vi "Inficon 32 Bit Data.vi"(7 "Gas Type":enum16{"Natural Gas", "Propane Gas"}(ring), 8 "Error In":errorcluster, 10 "Inficon Data Input":T3={"Gross Heating Value, Vol (Real, Dry)"=65535.0, "Nitrogen Component Normalized Mole % (Dry)"=8.0, "Methane Component Normalized Mole % (Dry)"=69.0, "Carbon Dioxide Component Normalized Mole % (Dry)"=65535.0, "Ethane Component Normalized Mole % (Dry)"=65.0, "Propane Component Normalized Mole % (Dry)"=8.0, "i-Pentane Component Normalized Mole % (Dry)"=14.0, "i-Butane Component Normalized Mole % (Dry)"=66.0, "n-Butane Component Normalized Mole % (Dry)"=8.0, "n-Pentane Component Normalized Mole % (Dry)"=0.0, "Hexane Component Normalized Mole % (Dry)"=0.0, "Heptane Component Normalized Mole % (Dry)"=0.0, "Gross Wobbe Index, Real(Dry)"=0.0, "Relative Density, Real(Dry)"=40.0, "Propylene Component Normalized Mole % (Dry)"=0.0, "C4 Olefins Component Normalized Mole % (Dry)"=0.0, "Water Component Normalized Mole % (Dry)"=0.0}, 11 "Modbus master in":refnum<class "Modbus Master.lvclass">=refnum) -> (0 "Error Out":errorcluster, 2 "Inficon Data Output":T3, 3 "Modbus master out":refnum<class "Modbus Master.lvclass">, 5 "Text Array":string[][](array[string]))   [LabVIEW 2023]
uses:
  Type Definitions/Inficon Data.ctl
  <vilib>/NI/Modbus Library/API/Master/Modbus Master.lvclass
  <vilib>/NI/Modbus Library/Transmission Data Unit/IP/IP Data Unit.lvclass
  <vilib>/NI/Modbus Library/Master Function Definition/Master Function Definition.lvclass
  <vilib>/NI/Modbus Library/Network Protocol/Network Master/TCP/TCP Master.lvclass
  Type Definitions/Inficon Modbus Addresses.ctl
  Type Definitions/Inficon Modbus Addresses LP.ctl
panel:
  in  "Density LP":T1=126 items=["Gross Heating Value (Dry)"=100, "Ethane"=102, "Propane"=104, "Proplyene"=106, "i-Butane"=108, "n-butane"=110, "C4 Olefins"=112, "Water"=114, "Gross Wobbe Index (Dry)"=124, "Relative Density (Dry)"=126]
  in  "Wobbe LP":T1=124 items=["Gross Heating Value (Dry)"=100, "Ethane"=102, "Propane"=104, "Proplyene"=106, "i-Butane"=108, "n-butane"=110, "C4 Olefins"=112, "Water"=114, "Gross Wobbe Index (Dry)"=124, "Relative Density (Dry)"=126]
  in  "Water":T1=114 items=["Gross Heating Value (Dry)"=100, "Ethane"=102, "Propane"=104, "Proplyene"=106, "i-Butane"=108, "n-butane"=110, "C4 Olefins"=112, "Water"=114, "Gross Wobbe Index (Dry)"=124, "Relative Density (Dry)"=126]
  in  "C4":T1=112 items=["Gross Heating Value (Dry)"=100, "Ethane"=102, "Propane"=104, "Proplyene"=106, "i-Butane"=108, "n-butane"=110, "C4 Olefins"=112, "Water"=114, "Gross Wobbe Index (Dry)"=124, "Relative Density (Dry)"=126]
  in  "n-Butane LP":T1=110 items=["Gross Heating Value (Dry)"=100, "Ethane"=102, "Propane"=104, "Proplyene"=106, "i-Butane"=108, "n-butane"=110, "C4 Olefins"=112, "Water"=114, "Gross Wobbe Index (Dry)"=124, "Relative Density (Dry)"=126]
  in  "i-Butane LP":T1=108 items=["Gross Heating Value (Dry)"=100, "Ethane"=102, "Propane"=104, "Proplyene"=106, "i-Butane"=108, "n-butane"=110, "C4 Olefins"=112, "Water"=114, "Gross Wobbe Index (Dry)"=124, "Relative Density (Dry)"=126]
  in  "Proplyene":T1=106 items=["Gross Heating Value (Dry)"=100, "Ethane"=102, "Propane"=104, "Proplyene"=106, "i-Butane"=108, "n-butane"=110, "C4 Olefins"=112, "Water"=114, "Gross Wobbe Index (Dry)"=124, "Relative Density (Dry)"=126]
  in  "Propane":T1=104 items=["Gross Heating Value (Dry)"=100, "Ethane"=102, "Propane"=104, "Proplyene"=106, "i-Butane"=108, "n-butane"=110, "C4 Olefins"=112, "Water"=114, "Gross Wobbe Index (Dry)"=124, "Relative Density (Dry)"=126]
  in  "Ethane":T1=102 items=["Gross Heating Value (Dry)"=100, "Ethane"=102, "Propane"=104, "Proplyene"=106, "i-Butane"=108, "n-butane"=110, "C4 Olefins"=112, "Water"=114, "Gross Wobbe Index (Dry)"=124, "Relative Density (Dry)"=126]
  in  "HHV LP":T1=100 items=["Gross Heating Value (Dry)"=100, "Ethane"=102, "Propane"=104, "Proplyene"=106, "i-Butane"=108, "n-butane"=110, "C4 Olefins"=112, "Water"=114, "Gross Wobbe Index (Dry)"=124, "Relative Density (Dry)"=126]
  in  "Density NG":T2=126 items=["Gross Heating Value (Dry)"=100, "Nitrogen"=102, "Methane"=104, "CO2"=106, "Ethane"=108, "Propane"=110, "i-Butane"=112, "n-Butane"=114, "i-Pentane"=116, "n-Pentane"=118, "Hexane"=120, "Heptane"=122, "Gross Wobbe Index (Dry)"=124, "Relative Density (Dry)"=126]
  in  "Wobbe NG":T2=124 items=["Gross Heating Value (Dry)"=100, "Nitrogen"=102, "Methane"=104, "CO2"=106, "Ethane"=108, "Propane"=110, "i-Butane"=112, "n-Butane"=114, "i-Pentane"=116, "n-Pentane"=118, "Hexane"=120, "Heptane"=122, "Gross Wobbe Index (Dry)"=124, "Relative Density (Dry)"=126]
  in  "Heptane":T2=122 items=["Gross Heating Value (Dry)"=100, "Nitrogen"=102, "Methane"=104, "CO2"=106, "Ethane"=108, "Propane"=110, "i-Butane"=112, "n-Butane"=114, "i-Pentane"=116, "n-Pentane"=118, "Hexane"=120, "Heptane"=122, "Gross Wobbe Index (Dry)"=124, "Relative Density (Dry)"=126]
  in  "Hexane":T2=120 items=["Gross Heating Value (Dry)"=100, "Nitrogen"=102, "Methane"=104, "CO2"=106, "Ethane"=108, "Propane"=110, "i-Butane"=112, "n-Butane"=114, "i-Pentane"=116, "n-Pentane"=118, "Hexane"=120, "Heptane"=122, "Gross Wobbe Index (Dry)"=124, "Relative Density (Dry)"=126]
  in  "n-Pentane":T2=118 items=["Gross Heating Value (Dry)"=100, "Nitrogen"=102, "Methane"=104, "CO2"=106, "Ethane"=108, "Propane"=110, "i-Butane"=112, "n-Butane"=114, "i-Pentane"=116, "n-Pentane"=118, "Hexane"=120, "Heptane"=122, "Gross Wobbe Index (Dry)"=124, "Relative Density (Dry)"=126]
  in  "i-Pentane":T2=116 items=["Gross Heating Value (Dry)"=100, "Nitrogen"=102, "Methane"=104, "CO2"=106, "Ethane"=108, "Propane"=110, "i-Butane"=112, "n-Butane"=114, "i-Pentane"=116, "n-Pentane"=118, "Hexane"=120, "Heptane"=122, "Gross Wobbe Index (Dry)"=124, "Relative Density (Dry)"=126]
  in  "n-Butane":T2=114 items=["Gross Heating Value (Dry)"=100, "Nitrogen"=102, "Methane"=104, "CO2"=106, "Ethane"=108, "Propane"=110, "i-Butane"=112, "n-Butane"=114, "i-Pentane"=116, "n-Pentane"=118, "Hexane"=120, "Heptane"=122, "Gross Wobbe Index (Dry)"=124, "Relative Density (Dry)"=126]
  in  "i-Butane":T2=112 items=["Gross Heating Value (Dry)"=100, "Nitrogen"=102, "Methane"=104, "CO2"=106, "Ethane"=108, "Propane"=110, "i-Butane"=112, "n-Butane"=114, "i-Pentane"=116, "n-Pentane"=118, "Hexane"=120, "Heptane"=122, "Gross Wobbe Index (Dry)"=124, "Relative Density (Dry)"=126]
  in  "Propane":T2=110 items=["Gross Heating Value (Dry)"=100, "Nitrogen"=102, "Methane"=104, "CO2"=106, "Ethane"=108, "Propane"=110, "i-Butane"=112, "n-Butane"=114, "i-Pentane"=116, "n-Pentane"=118, "Hexane"=120, "Heptane"=122, "Gross Wobbe Index (Dry)"=124, "Relative Density (Dry)"=126]
  in  "Ethane":T2=108 items=["Gross Heating Value (Dry)"=100, "Nitrogen"=102, "Methane"=104, "CO2"=106, "Ethane"=108, "Propane"=110, "i-Butane"=112, "n-Butane"=114, "i-Pentane"=116, "n-Pentane"=118, "Hexane"=120, "Heptane"=122, "Gross Wobbe Index (Dry)"=124, "Relative Density (Dry)"=126]
  in  "CO2":T2=106 items=["Gross Heating Value (Dry)"=100, "Nitrogen"=102, "Methane"=104, "CO2"=106, "Ethane"=108, "Propane"=110, "i-Butane"=112, "n-Butane"=114, "i-Pentane"=116, "n-Pentane"=118, "Hexane"=120, "Heptane"=122, "Gross Wobbe Index (Dry)"=124, "Relative Density (Dry)"=126]
  in  "CH4":T2=104 items=["Gross Heating Value (Dry)"=100, "Nitrogen"=102, "Methane"=104, "CO2"=106, "Ethane"=108, "Propane"=110, "i-Butane"=112, "n-Butane"=114, "i-Pentane"=116, "n-Pentane"=118, "Hexane"=120, "Heptane"=122, "Gross Wobbe Index (Dry)"=124, "Relative Density (Dry)"=126]
  in  "N":T2=102 items=["Gross Heating Value (Dry)"=100, "Nitrogen"=102, "Methane"=104, "CO2"=106, "Ethane"=108, "Propane"=110, "i-Butane"=112, "n-Butane"=114, "i-Pentane"=116, "n-Pentane"=118, "Hexane"=120, "Heptane"=122, "Gross Wobbe Index (Dry)"=124, "Relative Density (Dry)"=126]
  in  "HHV NG":T2=100 items=["Gross Heating Value (Dry)"=100, "Nitrogen"=102, "Methane"=104, "CO2"=106, "Ethane"=108, "Propane"=110, "i-Butane"=112, "n-Butane"=114, "i-Pentane"=116, "n-Pentane"=118, "Hexane"=120, "Heptane"=122, "Gross Wobbe Index (Dry)"=124, "Relative Density (Dry)"=126]
  # "Propane Gas"
  # "Natural Gas"
  # "Natural Gas"
  # "Propane"
  # "Natural Gas"
  # "Propane"
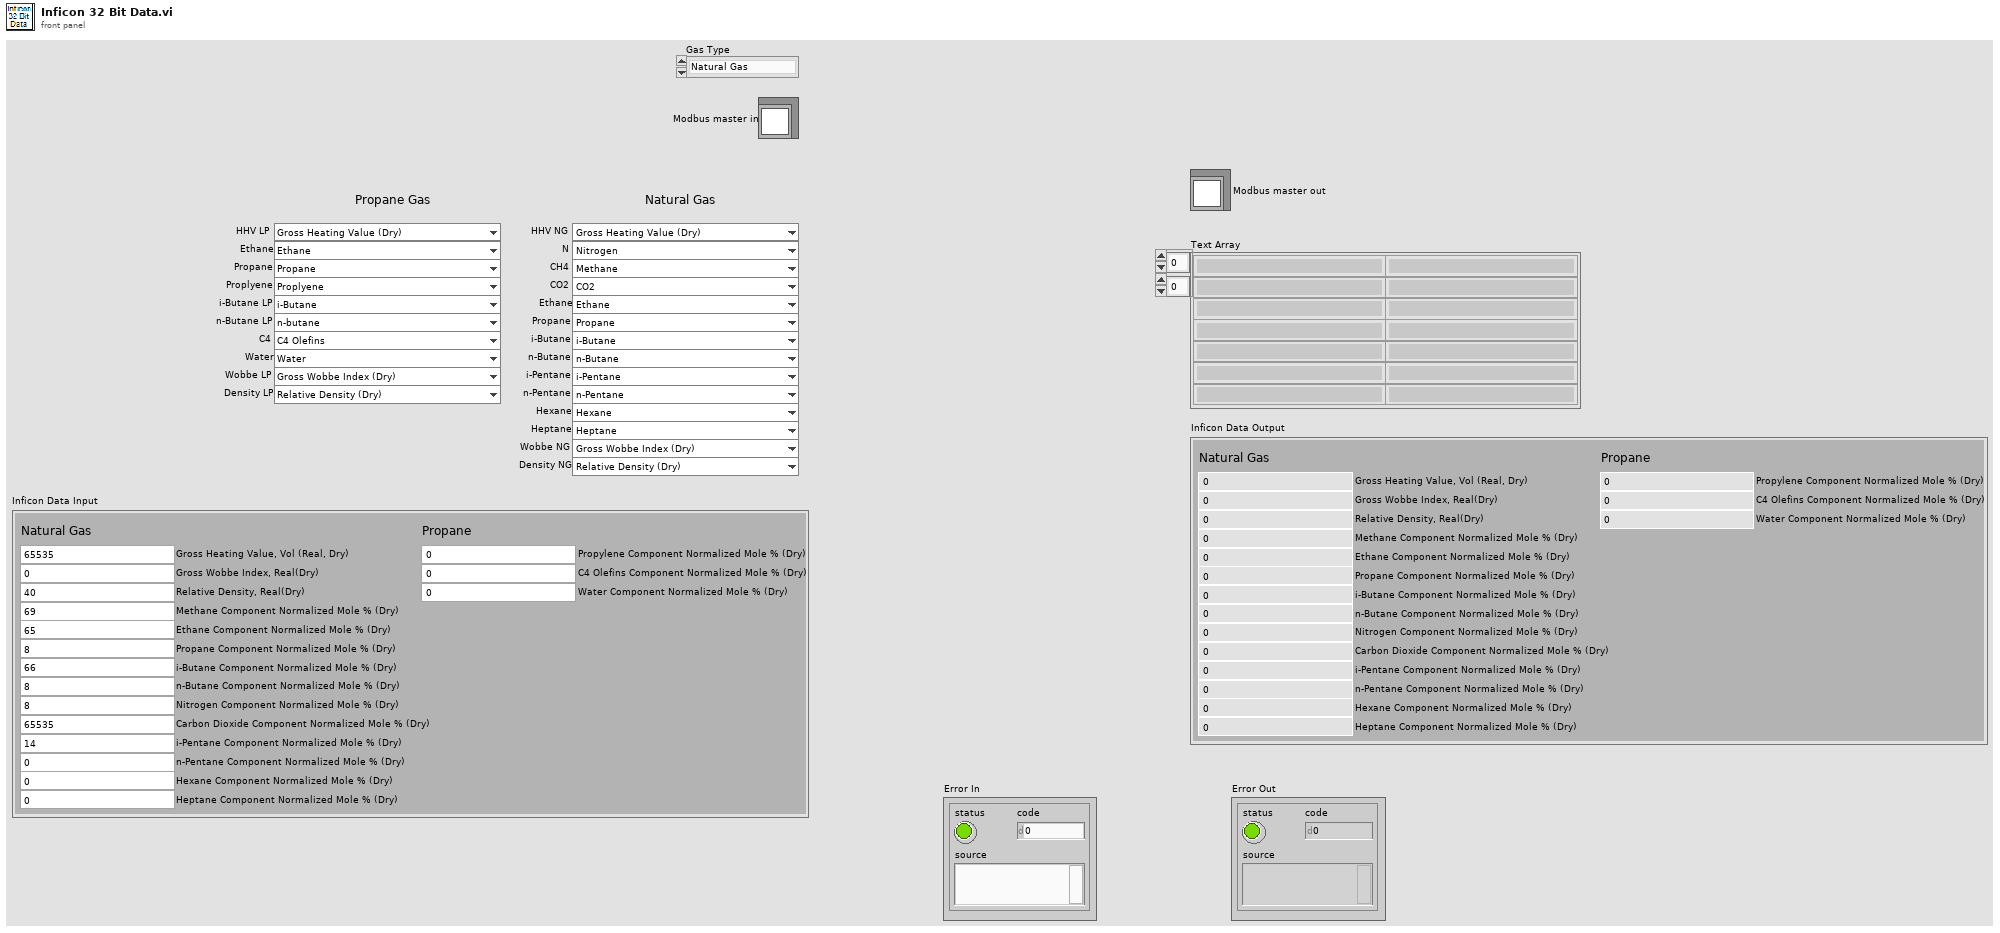
[diagram p1: front panel]
types:
  T1 = typedef "Inficon Modbus Addresses LP.ctl" = u16
  T2 = typedef "Inficon Modbus Addresses.ctl" = u16
  T3 = typedef "Inficon Data.ctl" = cluster{"Gross Heating Value, Vol (Real, Dry)":dbl, "Nitrogen Component Normalized Mole % (Dry)":dbl, "Methane Component Normalized Mole % (Dry)":dbl, "Carbon Dioxide Component Normalized Mole % (Dry)":dbl, "Ethane Component Normalized Mole % (Dry)":dbl, "Propane Component Normalized Mole % (Dry)":dbl, "i-Pentane Component Normalized Mole % (Dry)":dbl, "i-Butane Component Normalized Mole % (Dry)":dbl, "n-Butane Component Normalized Mole % (Dry)":dbl, "n-Pentane Component Normalized Mole % (Dry)":dbl, "Hexane Component Normalized Mole % (Dry)":dbl, "Heptane Component Normalized Mole % (Dry)":dbl, "Gross Wobbe Index, Real(Dry)":dbl, "Relative Density, Real(Dry)":dbl, "Propylene Component Normalized Mole % (Dry)":dbl, "C4 Olefins Component Normalized Mole % (Dry)":dbl, "Water Component Normalized Mole % (Dry)":dbl}
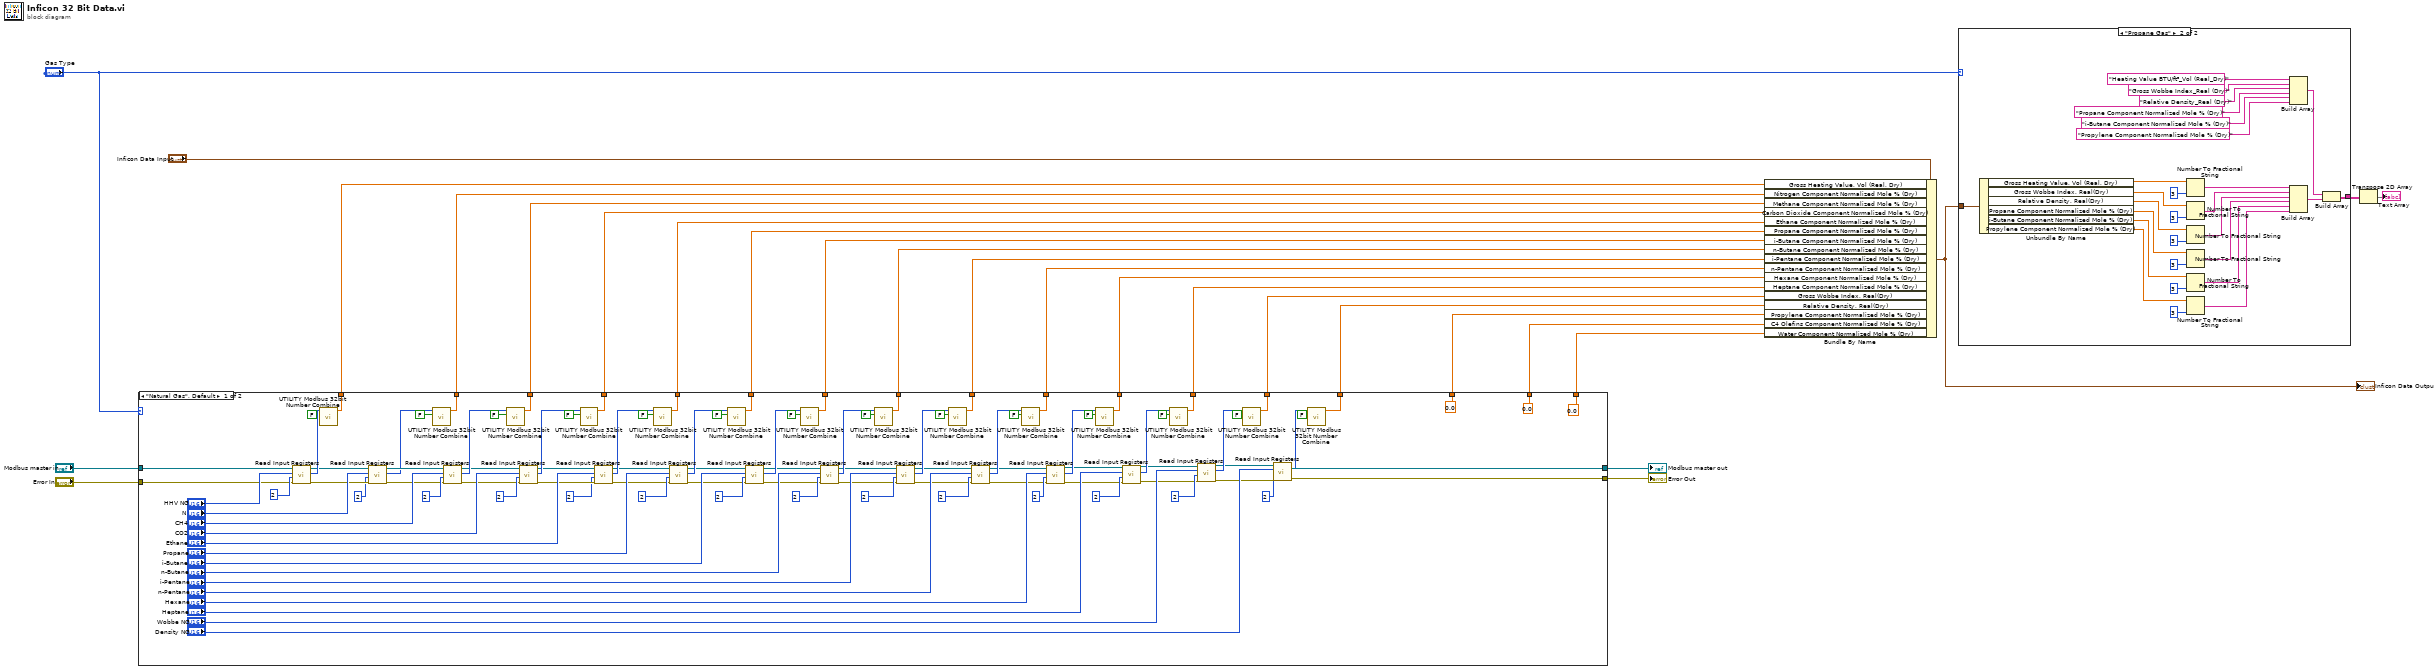
[diagram p0: block diagram]
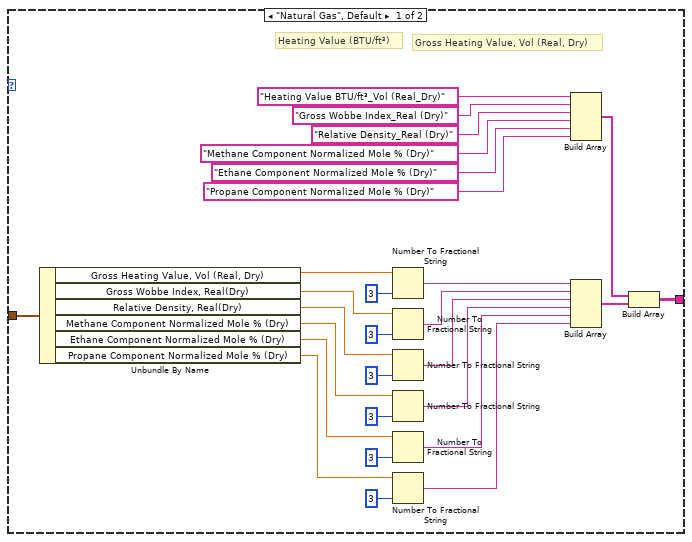
[diagram p2: hidden frame]
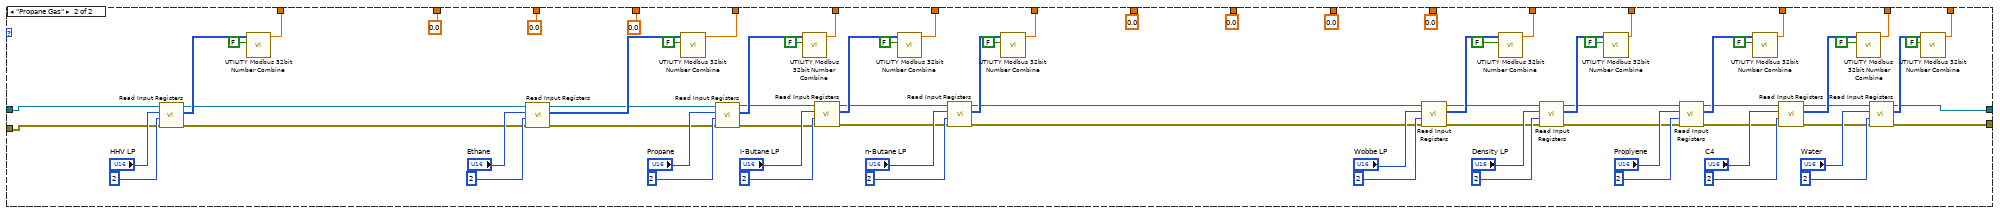
[diagram p3: hidden frame]
diagram:
  n1 = case shown="\"Natural Gas\", Default" "Gas Type" {
    tunnel: [w129 w202] -> w25
    tunnel: [w128 sgl 0.0 ("Data")] -> w24
    tunnel: [w127 sgl 0.0 ("Data")] -> w23
    tunnel: [w126 sgl 0.0 ("Data")] -> w22
    tunnel: [w125 w194] -> w21
    tunnel: [w124 sgl 0.0 ("Data")] -> w20
    tunnel: [w123 w190] -> w19
    tunnel: [w122 w184] -> w18
    tunnel: [w121 w179] -> w17
    tunnel: [w120 sgl 0.0 ("Data")] -> w16
    tunnel: "Modbus master in" -> [w111 w203]
    tunnel: "Error In" -> [w107 w204]
    tunnel: [w102 w130] -> w13
    tunnel: [w101 w131] -> w12
    tunnel: [w100 sgl 0.0 ("Data")] -> w11
    tunnel: [w99 sgl 0.0 ("Data")] -> w10
    tunnel: [w98 w171] -> w9
    tunnel: [w97 w165] -> w8
    tunnel: [0.0 ("Propylene Component Normalized Mole % (Dry)") w160] -> w4
    tunnel: [0.0 ("Propylene Component Normalized Mole % (Dry)") w151] -> w3
    tunnel: [0.0 ("Propylene Component Normalized Mole % (Dry)") w150] -> w2
    frame "Natural Gas", Default {
      n2 = call-dynamic "Read Input Registers.vi"("error in"=w107, "number of inputs"=u16 2 ("Quantity"), "starting address"="HHV NG", "Modbus master in"=w111) -> ("error out"=w103:errorcluster, "register values"=w108:u16[], "Modbus master out"=w105:refnum<class "Modbus Master.lvclass">)  [unwired: 5 in]
      n3 = call "UTILITY Modbus 32bit Number Combine.vi"("Swap Words"=FALSE, "Holding Registers"=w108) -> ("Data"=w129:sgl)  [unwired: 8 in, 1 out]
      n4 = call-dynamic "Read Input Registers.vi"("error in"=w103, "number of inputs"=u16 2 ("Quantity"), "starting address"="N", "Modbus master in"=w105) -> ("error out"=w58:errorcluster, "register values"=w59:u16[], "Modbus master out"=w60:refnum<class "Modbus Master.lvclass">)  [unwired: 5 in]
      n5 = call "UTILITY Modbus 32bit Number Combine.vi"("Swap Words"=FALSE, "Holding Registers"=w59) -> ("Data"=w128:sgl)  [unwired: 8 in, 1 out]
      n6 = call-dynamic "Read Input Registers.vi"("error in"=w58, "number of inputs"=u16 2 ("Quantity"), "starting address"="CH4", "Modbus master in"=w60) -> ("error out"=w85:errorcluster, "register values"=w91:u16[], "Modbus master out"=w87:refnum<class "Modbus Master.lvclass">)  [unwired: 5 in]
      n7 = call "UTILITY Modbus 32bit Number Combine.vi"("Swap Words"=FALSE, "Holding Registers"=w91) -> ("Data"=w127:sgl)  [unwired: 8 in, 1 out]
      n8 = call-dynamic "Read Input Registers.vi"("error in"=w85, "number of inputs"=u16 2 ("Quantity"), "starting address"="CO2", "Modbus master in"=w87) -> ("error out"=w84:errorcluster, "register values"=w90:u16[], "Modbus master out"=w86:refnum<class "Modbus Master.lvclass">)  [unwired: 5 in]
      n9 = call "UTILITY Modbus 32bit Number Combine.vi"("Swap Words"=FALSE, "Holding Registers"=w90) -> ("Data"=w126:sgl)  [unwired: 8 in, 1 out]
      n10 = call-dynamic "Read Input Registers.vi"("error in"=w84, "number of inputs"=u16 2 ("Quantity"), "starting address"="Ethane", "Modbus master in"=w86) -> ("error out"=w73:errorcluster, "register values"=w88:u16[], "Modbus master out"=w68:refnum<class "Modbus Master.lvclass">)  [unwired: 5 in]
      n11 = call "UTILITY Modbus 32bit Number Combine.vi"("Swap Words"=FALSE, "Holding Registers"=w88) -> ("Data"=w125:sgl)  [unwired: 8 in, 1 out]
      n12 = call-dynamic "Read Input Registers.vi"("error in"=w73, "number of inputs"=u16 2 ("Quantity"), "starting address"="Propane", "Modbus master in"=w68) -> ("error out"=w72:errorcluster, "register values"=w83:u16[], "Modbus master out"=w67:refnum<class "Modbus Master.lvclass">)  [unwired: 5 in]
      n13 = call "UTILITY Modbus 32bit Number Combine.vi"("Swap Words"=FALSE, "Holding Registers"=w83) -> ("Data"=w123:sgl)  [unwired: 8 in, 1 out]
      n14 = call-dynamic "Read Input Registers.vi"("error in"=w72, "number of inputs"=u16 2 ("Quantity"), "starting address"="i-Butane", "Modbus master in"=w67) -> ("error out"=w71:errorcluster, "register values"=w80:u16[], "Modbus master out"=w66:refnum<class "Modbus Master.lvclass">)  [unwired: 5 in]
      n15 = call "UTILITY Modbus 32bit Number Combine.vi"("Swap Words"=FALSE, "Holding Registers"=w80) -> ("Data"=w122:sgl)  [unwired: 8 in, 1 out]
      n16 = call-dynamic "Read Input Registers.vi"("error in"=w71, "number of inputs"=u16 2 ("Quantity"), "starting address"="n-Butane", "Modbus master in"=w66) -> ("error out"=w70:errorcluster, "register values"=w79:u16[], "Modbus master out"=w65:refnum<class "Modbus Master.lvclass">)  [unwired: 5 in]
      n17 = call "UTILITY Modbus 32bit Number Combine.vi"("Swap Words"=FALSE, "Holding Registers"=w79) -> ("Data"=w121:sgl)  [unwired: 8 in, 1 out]
      n18 = call-dynamic "Read Input Registers.vi"("error in"=w70, "number of inputs"=u16 2 ("Quantity"), "starting address"="i-Pentane", "Modbus master in"=w65) -> ("error out"=w69:errorcluster, "register values"=w76:u16[], "Modbus master out"=w64:refnum<class "Modbus Master.lvclass">)  [unwired: 5 in]
      n19 = call "UTILITY Modbus 32bit Number Combine.vi"("Swap Words"=FALSE, "Holding Registers"=w76) -> ("Data"=w120:sgl)  [unwired: 8 in, 1 out]
      n20 = call-dynamic "Read Input Registers.vi"("error in"=w69, "number of inputs"=u16 2 ("Quantity"), "starting address"="n-Pentane", "Modbus master in"=w64) -> ("error out"=w38:errorcluster, "register values"=w75:u16[], "Modbus master out"=w31:refnum<class "Modbus Master.lvclass">)  [unwired: 5 in]
      n21 = call "UTILITY Modbus 32bit Number Combine.vi"("Swap Words"=FALSE, "Holding Registers"=w75) -> ("Data"=w124:sgl)  [unwired: 8 in, 1 out]
      n22 = call-dynamic "Read Input Registers.vi"("error in"=w38, "number of inputs"=u16 2 ("Quantity"), "starting address"="Hexane", "Modbus master in"=w31) -> ("error out"=w37:errorcluster, "register values"=w47:u16[], "Modbus master out"=w32:refnum<class "Modbus Master.lvclass">)  [unwired: 5 in]
      n23 = call "UTILITY Modbus 32bit Number Combine.vi"("Swap Words"=FALSE, "Holding Registers"=w47) -> ("Data"=w100:sgl)  [unwired: 8 in, 1 out]
      n24 = call-dynamic "Read Input Registers.vi"("error in"=w37, "number of inputs"=u16 2 ("Quantity"), "starting address"="Heptane", "Modbus master in"=w32) -> ("error out"=w36:errorcluster, "register values"=w46:u16[], "Modbus master out"=w33:refnum<class "Modbus Master.lvclass">)  [unwired: 5 in]
      n25 = call "UTILITY Modbus 32bit Number Combine.vi"("Swap Words"=FALSE, "Holding Registers"=w46) -> ("Data"=w99:sgl)  [unwired: 8 in, 1 out]
      n26 = call-dynamic "Read Input Registers.vi"("error in"=w36, "number of inputs"=u16 2 ("Quantity"), "starting address"="Wobbe NG", "Modbus master in"=w33) -> ("error out"=w35:errorcluster, "register values"=w41:u16[], "Modbus master out"=w34:refnum<class "Modbus Master.lvclass">)  [unwired: 5 in]
      n27 = call "UTILITY Modbus 32bit Number Combine.vi"("Swap Words"=FALSE, "Holding Registers"=w41) -> ("Data"=w98:sgl)  [unwired: 8 in, 1 out]
      n28 = call-dynamic "Read Input Registers.vi"("error in"=w35, "number of inputs"=u16 2 ("Quantity"), "starting address"="Density NG", "Modbus master in"=w34) -> ("error out"=w102:errorcluster, "register values"=w30:u16[], "Modbus master out"=w101:refnum<class "Modbus Master.lvclass">)  [unwired: 5 in]
      n29 = call "UTILITY Modbus 32bit Number Combine.vi"("Swap Words"=FALSE, "Holding Registers"=w30) -> ("Data"=w97:sgl)  [unwired: 8 in, 1 out]
    }
    frame "Propane Gas" {
      n30 = call-dynamic "Read Input Registers.vi"("error in"=w204, "number of inputs"=u16 2 ("Quantity"), "starting address"="HHV LP", "Modbus master in"=w203) -> ("error out"=w149:errorcluster, "register values"=w207:u16[], "Modbus master out"=w148:refnum<class "Modbus Master.lvclass">)  [unwired: 5 in]
      n31 = call "UTILITY Modbus 32bit Number Combine.vi"("Swap Words"=FALSE, "Holding Registers"=w207) -> ("Data"=w202:sgl)  [unwired: 8 in, 1 out]
      n32 = call-dynamic "Read Input Registers.vi"("error in"=w149, "number of inputs"=u16 2 ("Quantity"), "starting address"="Ethane", "Modbus master in"=w148) -> ("error out"=w147:errorcluster, "register values"=w196:u16[], "Modbus master out"=w144:refnum<class "Modbus Master.lvclass">)  [unwired: 5 in]
      n33 = call "UTILITY Modbus 32bit Number Combine.vi"("Swap Words"=FALSE, "Holding Registers"=w196) -> ("Data"=w194:sgl)  [unwired: 8 in, 1 out]
      n34 = call-dynamic "Read Input Registers.vi"("error in"=w147, "number of inputs"=u16 2 ("Quantity"), "starting address"="Propane", "Modbus master in"=w144) -> ("error out"=w146:errorcluster, "register values"=w193:u16[], "Modbus master out"=w145:refnum<class "Modbus Master.lvclass">)  [unwired: 5 in]
      n35 = call "UTILITY Modbus 32bit Number Combine.vi"("Swap Words"=FALSE, "Holding Registers"=w193) -> ("Data"=w190:sgl)  [unwired: 8 in, 1 out]
      n36 = call-dynamic "Read Input Registers.vi"("error in"=w146, "number of inputs"=u16 2 ("Quantity"), "starting address"="i-Butane LP", "Modbus master in"=w145) -> ("error out"=w143:errorcluster, "register values"=w188:u16[], "Modbus master out"=w142:refnum<class "Modbus Master.lvclass">)  [unwired: 5 in]
      n37 = call "UTILITY Modbus 32bit Number Combine.vi"("Swap Words"=FALSE, "Holding Registers"=w188) -> ("Data"=w184:sgl)  [unwired: 8 in, 1 out]
      n38 = call-dynamic "Read Input Registers.vi"("error in"=w143, "number of inputs"=u16 2 ("Quantity"), "starting address"="n-Butane LP", "Modbus master in"=w142) -> ("error out"=w141:errorcluster, "register values"=w181:u16[], "Modbus master out"=w140:refnum<class "Modbus Master.lvclass">)  [unwired: 5 in]
      n39 = call "UTILITY Modbus 32bit Number Combine.vi"("Swap Words"=FALSE, "Holding Registers"=w181) -> ("Data"=w179:sgl)  [unwired: 8 in, 1 out]
      n40 = call-dynamic "Read Input Registers.vi"("error in"=w141, "number of inputs"=u16 2 ("Quantity"), "starting address"="Wobbe LP", "Modbus master in"=w140) -> ("error out"=w139:errorcluster, "register values"=w172:u16[], "Modbus master out"=w138:refnum<class "Modbus Master.lvclass">)  [unwired: 5 in]
      n41 = call "UTILITY Modbus 32bit Number Combine.vi"("Swap Words"=FALSE, "Holding Registers"=w172) -> ("Data"=w171:sgl)  [unwired: 8 in, 1 out]
      n42 = call-dynamic "Read Input Registers.vi"("error in"=w139, "number of inputs"=u16 2 ("Quantity"), "starting address"="Density LP", "Modbus master in"=w138) -> ("error out"=w137:errorcluster, "register values"=w169:u16[], "Modbus master out"=w136:refnum<class "Modbus Master.lvclass">)  [unwired: 5 in]
      n43 = call "UTILITY Modbus 32bit Number Combine.vi"("Swap Words"=FALSE, "Holding Registers"=w169) -> ("Data"=w165:sgl)  [unwired: 8 in, 1 out]
      n44 = call-dynamic "Read Input Registers.vi"("error in"=w137, "number of inputs"=u16 2 ("Quantity"), "starting address"="Proplyene", "Modbus master in"=w136) -> ("error out"=w134:errorcluster, "register values"=w162:u16[], "Modbus master out"=w135:refnum<class "Modbus Master.lvclass">)  [unwired: 5 in]
      n45 = call "UTILITY Modbus 32bit Number Combine.vi"("Swap Words"=FALSE, "Holding Registers"=w162) -> ("Data"=w160:sgl)  [unwired: 8 in, 1 out]
      n46 = call-dynamic "Read Input Registers.vi"("error in"=w134, "number of inputs"=u16 2 ("Quantity"), "starting address"="C4", "Modbus master in"=w135) -> ("error out"=w133:errorcluster, "register values"=w159:u16[], "Modbus master out"=w132:refnum<class "Modbus Master.lvclass">)  [unwired: 5 in]
      n47 = call "UTILITY Modbus 32bit Number Combine.vi"("Swap Words"=FALSE, "Holding Registers"=w159) -> ("Data"=w151:sgl)  [unwired: 8 in, 1 out]
      n48 = call-dynamic "Read Input Registers.vi"("error in"=w133, "number of inputs"=u16 2 ("Quantity"), "starting address"="Water", "Modbus master in"=w132) -> ("error out"=w130:errorcluster, "register values"=w153:u16[], "Modbus master out"=w131:refnum<class "Modbus Master.lvclass">)  [unwired: 5 in]
      n49 = call "UTILITY Modbus 32bit Number Combine.vi"("Swap Words"=FALSE, "Holding Registers"=w153) -> ("Data"=w150:sgl)  [unwired: 8 in, 1 out]
    }
  }
  "Error Out" <- w13
  "Modbus master out" <- w12
  n50 = Bundle By Name(cluster="Inficon Data Input", "Gross Heating Value, Vol (Real, Dry)"=w25, "Nitrogen Component Normalized Mole % (Dry)"=w24, "Methane Component Normalized Mole % (Dry)"=w23, "Carbon Dioxide Component Normalized Mole % (Dry)"=w22, "Ethane Component Normalized Mole % (Dry)"=w21, "Propane Component Normalized Mole % (Dry)"=w19, "i-Butane Component Normalized Mole % (Dry)"=w18, "n-Butane Component Normalized Mole % (Dry)"=w17, "i-Pentane Component Normalized Mole % (Dry)"=w16, "n-Pentane Component Normalized Mole % (Dry)"=w20, "Hexane Component Normalized Mole % (Dry)"=w11, "Heptane Component Normalized Mole % (Dry)"=w10, "Gross Wobbe Index, Real(Dry)"=w9, "Relative Density, Real(Dry)"=w8, "Propylene Component Normalized Mole % (Dry)"=w4, "C4 Olefins Component Normalized Mole % (Dry)"=w3, "Water Component Normalized Mole % (Dry)"=w2) -> (w7:T3)
  "Inficon Data Output" <- w7
  n51 = case shown="\"Propane Gas\"" "Gas Type" {
    tunnel: w7 -> [w236 w237]
    tunnel: [w229 w238] -> w6
    frame "Natural Gas", Default {
      # "Gross Heating Value, Vol (Real, Dry)"
      # "Heating Value (BTU/ft³)"
      n52 = Unbundle By Name(w236) -> ("Gross Heating Value, Vol (Real, Dry)"=w235:dbl, "Gross Wobbe Index, Real(Dry)"=w223:dbl, "Relative Density, Real(Dry)"=w222:dbl, "Methane Component Normalized Mole % (Dry)"=w221:dbl, "Ethane Component Normalized Mole % (Dry)"=w220:dbl, "Propane Component Normalized Mole % (Dry)"=w219:dbl)
      n53 = Number To Fractional String(number=w235, precision (6)=i16 3) -> (F-format string=w232:string)  [unwired: 2 in]
      n54 = Number To Fractional String(number=w223, precision (6)=i16 3) -> (F-format string=w218:string)  [unwired: 2 in]
      n55 = Number To Fractional String(number=w222, precision (6)=i16 3) -> (F-format string=w217:string)  [unwired: 2 in]
      n56 = Number To Fractional String(number=w221, precision (6)=i16 3) -> (F-format string=w216:string)  [unwired: 2 in]
      n57 = Number To Fractional String(number=w220, precision (6)=i16 3) -> (F-format string=w215:string)  [unwired: 2 in]
      n58 = Number To Fractional String(number=w219, precision (6)=i16 3) -> (F-format string=w214:string)  [unwired: 2 in]
      n59 = Build Array("Heating Value BTU/ft³_Vol (Real_Dry)", "Gross Wobbe Index_Real (Dry)", "Relative Density_Real (Dry)", "Methane Component Normalized Mole % (Dry)", "Ethane Component Normalized Mole % (Dry)", "Propane Component Normalized Mole % (Dry)") -> (w231:string[])
      n60 = Build Array(w232, w218, w217, w216, w215, w214) -> (w230:string[])
      n61 = Build Array(w231, w230) -> (w229:string[][])
    }
    frame "Propane Gas" {
      n62 = Unbundle By Name(w237) -> ("Gross Heating Value, Vol (Real, Dry)"=w264:dbl, "Gross Wobbe Index, Real(Dry)"=w260:dbl, "Relative Density, Real(Dry)"=w259:dbl, "Propane Component Normalized Mole % (Dry)"=w258:dbl, "i-Butane Component Normalized Mole % (Dry)"=w257:dbl, "Propylene Component Normalized Mole % (Dry)"=w256:dbl)
      n63 = Number To Fractional String(number=w264, precision (6)=i16 3) -> (F-format string=w263:string)  [unwired: 2 in]
      n64 = Number To Fractional String(number=w260, precision (6)=i16 3) -> (F-format string=w255:string)  [unwired: 2 in]
      n65 = Number To Fractional String(number=w259, precision (6)=i16 3) -> (F-format string=w254:string)  [unwired: 2 in]
      n66 = Number To Fractional String(number=w258, precision (6)=i16 3) -> (F-format string=w253:string)  [unwired: 2 in]
      n67 = Number To Fractional String(number=w257, precision (6)=i16 3) -> (F-format string=w252:string)  [unwired: 2 in]
      n68 = Number To Fractional String(number=w256, precision (6)=i16 3) -> (F-format string=w251:string)  [unwired: 2 in]
      n69 = Build Array("Heating Value BTU/ft³_Vol (Real_Dry)", "Gross Wobbe Index_Real (Dry)", "Relative Density_Real (Dry)", "Propane Component Normalized Mole % (Dry)", "i-Butane Component Normalized Mole % (Dry)", "Propylene Component Normalized Mole % (Dry)") -> (w262:string[])
      n70 = Build Array(w263, w255, w254, w253, w252, w251) -> (w261:string[])
      n71 = Build Array(w262, w261) -> (w238:string[][])
    }
  }
  n72 = Transpose 2D Array(2D array=w6) -> (transposed array=→"Text Array":string[][])
